vi "Panel.vi"(11 "Item Summary in":refnum<class "Item Summary.lvclass">) -> ()   [LabVIEW 2020, in "Item Summary.lvclass"]
uses:
  Item Summary.lvclass
  C:/dev/LabVIEW/lv-oopanel/OOPanel/Panel/Panel.lvclass
  Item/Item.lvclass
  Item Summary.lvclass/Item Summary.ctl
  Workstation/Workstation.lvclass
  lv-oopanel/OOPanel/Panel/Panel.lvclass
panel:
  out "Item":refnum<class "Item.lvclass">
  out "# Stations":i32
  out "Craft Time":dbl format="%<%M:%S>t"
  out "Item Name":string
  in  "Craft At":string(combo)
  out "Qty":dbl
  out "Item Picture":picture
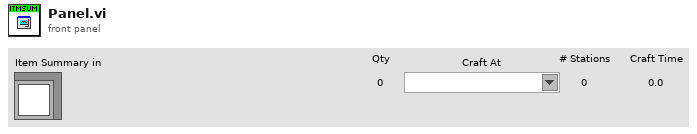
[diagram p1: front panel]
types:
  T1 = typedef "OOPanel.lvlib/Panel.lvclass/Panel Events.ctl" = cluster{"Visbility":refnum<user-event>, "Close":refnum<user-event>}
  T2 = typedef "Item.lvclass/Craft Station.ctl" = cluster{"Station":refnum<class "Workstation.lvclass">, "Craft Time":dbl, "Qty Made":dbl}
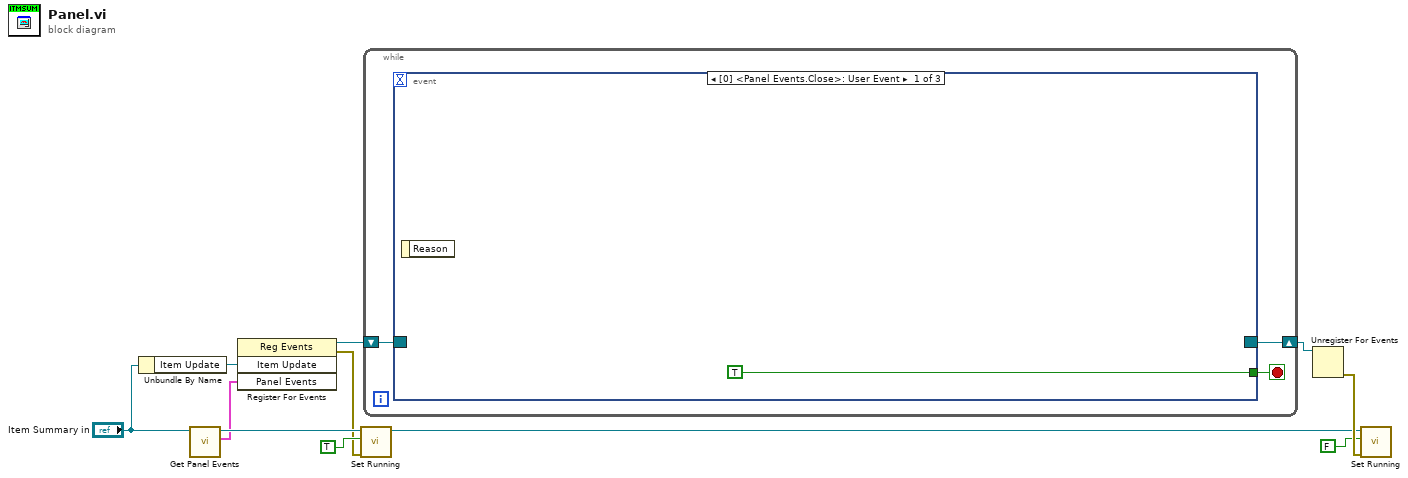
[diagram p0: block diagram]
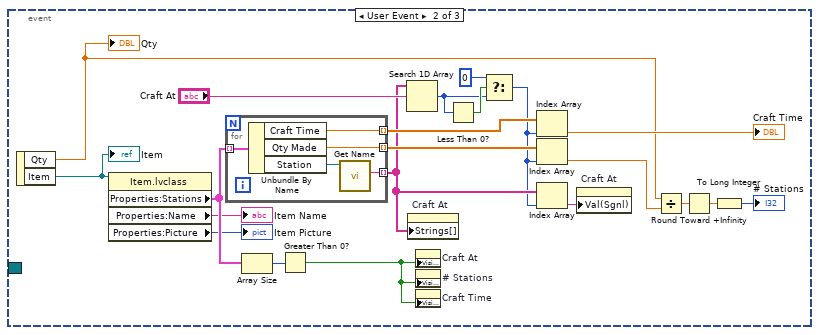
[diagram p2: hidden frame]
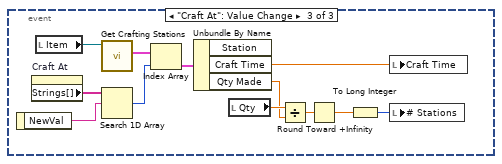
[diagram p3: hidden frame]
diagram:
  n1 = Unbundle By Name("Item Summary in") -> ("Item Update"=w4:refnum<user-event>)
  n2 = call "Get Panel Events.vi"("Panel in"="Item Summary in") -> ("Panel Events"=w3:T1, "Panel out"=w7:refnum<class "Item Summary.lvclass">)  [unwired: 8 in, 1 out]
  n3 = register-events(w4, w3) -> (reference out=w2:refnum<event-registration>, error out=w1:errorcluster)  [unwired: 2 in]
  n4 = call "Set Running.vi"("error in (no error)"=w1, "Running"=TRUE, "Panel in"=w7) -> ("Panel out"=w8:refnum<class "Item Summary.lvclass">)  [unwired: 7 in, 1 out]
  n5 = while {
    shift-right: [w13] -> w9
    shift-left: w2 -> [w14]
    stop <- w12 stop-if-true
    n6 = event shown="[0] <Panel Events.Close>: User Event" {
      selector: w14 -> [_ _ _]
      dyn-events: [_ _ _] -> w13
      timeout: _ -> [_ _ _]
      tunnel: [TRUE _ _] -> w12
      event User Event {
        n7 = event-data() -> ()  [unwired: 1 in, 1 out]
      }
      event User Event {
        n8 = event-data() -> ("Qty"=w16:dbl, "Item"=w17:refnum<class "Item.lvclass">)  [unwired: 1 in]
        "Qty" <- w16
        "Item" <- w17
        n9 = property class="Item.lvclass"(reference=w17) -> ("Properties:Stations"=w33:T2[], "Properties:Name"=→"Item Name":string, "Properties:Picture"=→"Item Picture":picture)  [unwired: 1 in, 2 out]
        n10 = for {
          tunnel: w33 -> [w41] mode=indexing
          tunnel: [w39] -> w30 mode=indexing
          tunnel: [w38] -> w29 mode=indexing
          tunnel: [w37] -> w21 mode=indexing
          n11 = Unbundle By Name(w41) -> ("Craft Time"=w39:dbl, "Qty Made"=w38:dbl, "Station"=w40:refnum<class "Workstation.lvclass">)
          n12 = call "Get Name.vi"("Workstation in"=w40) -> ("Name"=w37:string)  [unwired: 8 in, 2 out]
        }
        n13 = Array Size(array=w33) -> (size(s)=w34:i32)
        n14 = Greater Than 0?(x=w34) -> (x > 0?=w35:bool)
        n15 = Search 1D Array(1D array=w21, element="Craft At") -> (index of element=w22:i32)  [unwired: 1 in]
        n16 = property on="Craft At" class="CmbBox"("Strings[]"=w21) -> ()  [unwired: 2 in, 2 out]
        n17 = property on="Craft At" class="CmbBox"("Visible"=w35) -> ()  [unwired: 2 in, 2 out]
        n18 = property on="# Stations" class="DigNum (strict)"("Visible"=w35) -> ()  [unwired: 2 in, 2 out]
        n19 = property on="Craft Time" class="DigNum (strict)"("Visible"=w35) -> ()  [unwired: 2 in, 2 out]
        n20 = Less Than 0?(x=w22) -> (x < 0?=w23:bool)
        n21 = Select(t=0 ("f"), s=w23, f=w22) -> (s? t:f=w20:i32)
        n22 = Index Array(array=w30, index=w20) -> (element=→"Craft Time":dbl)
        n23 = Index Array(array=w29, index=w20) -> (element=w26:dbl)
        n24 = Index Array(array=w21, index=w20) -> (element=w19:string)
        n25 = property on="Craft At" class="CmbBox"("Val(Sgnl)"=w19) -> ()  [unwired: 2 in, 2 out]
        n26 = Divide(x=w16, y=w26) -> (x/y=w25:dbl)
        n27 = Round Toward +Infinity(x=w25) -> (ceil(x): smallest int >= x=w24:dbl)
        n28 = To Long Integer(number=w24) -> (32bit integer=→"# Stations":i32)
      }
      event "Craft At": Value Change {
        n29 = event-data() -> ("NewVal"=w52:string)  [unwired: 1 in]
        n30 = property on="Craft At" class="CmbBox"() -> ("Strings[]"=w53:string[])  [unwired: 2 in, 2 out]
        n31 = local read "Item"() -> (w48:refnum<class "Item.lvclass">)
        n32 = call-dynamic "Get Crafting Stations.vi"("Item in"=w48) -> ("Stations"=w51:T2[])  [unwired: 8 in, 2 out]
        n33 = Search 1D Array(1D array=w53, element=w52) -> (index of element=w50:i32)  [unwired: 1 in]
        n34 = Index Array(array=w51, index=w50) -> (element=w49:T2)
        n35 = Unbundle By Name(w49) -> ("Craft Time"=w42:dbl, "Qty Made"=w46:dbl)  [unwired: 1 out]
        n36 = local read "Qty"() -> (w47:dbl)
        n37 = Divide(x=w47, y=w46) -> (x/y=w45:dbl)
        n38 = Round Toward +Infinity(x=w45) -> (ceil(x): smallest int >= x=w44:dbl)
        n39 = To Long Integer(number=w44) -> (32bit integer=w43:i32)
        n40 = local write "Craft Time"(w42) -> ()
        n41 = local write "# Stations"(w43) -> ()
      }
    }
  }
  n42 = Unregister For Events(event registration refnum=w9) -> (error out=w11:errorcluster)  [unwired: 1 in]
  n43 = call "Set Running.vi"("error in (no error)"=w11, "Running"=FALSE, "Panel in"=w8) -> ()  [unwired: 7 in, 2 out]
